vi "pumpPIDantiWindup_Filter.vi"(4 "Saturation U":dbl, 6 "Saturation M":dbl, 7 "Reset":bool, 8 "PID Gains":cluster{"Kp":dbl, "Kd":dbl, "Ki":dbl, "Ts":dbl}={"Kp"=0.0, "Kd"=0.0, "Ki"=0.0, "Ts"=1.0}, 10 "Feedback":dbl, 11 "Reference":dbl) -> (3 "Control":dbl)   [LabVIEW 2016]
uses:
  <vilib>/ptbypt/NI_PtbyPt.lvlib
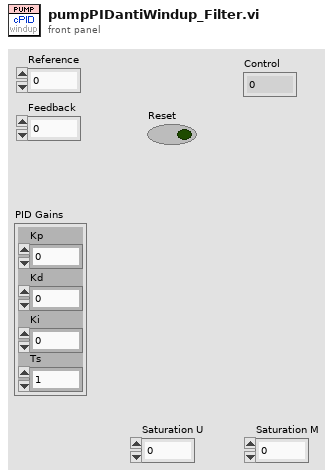
[diagram p1: front panel]
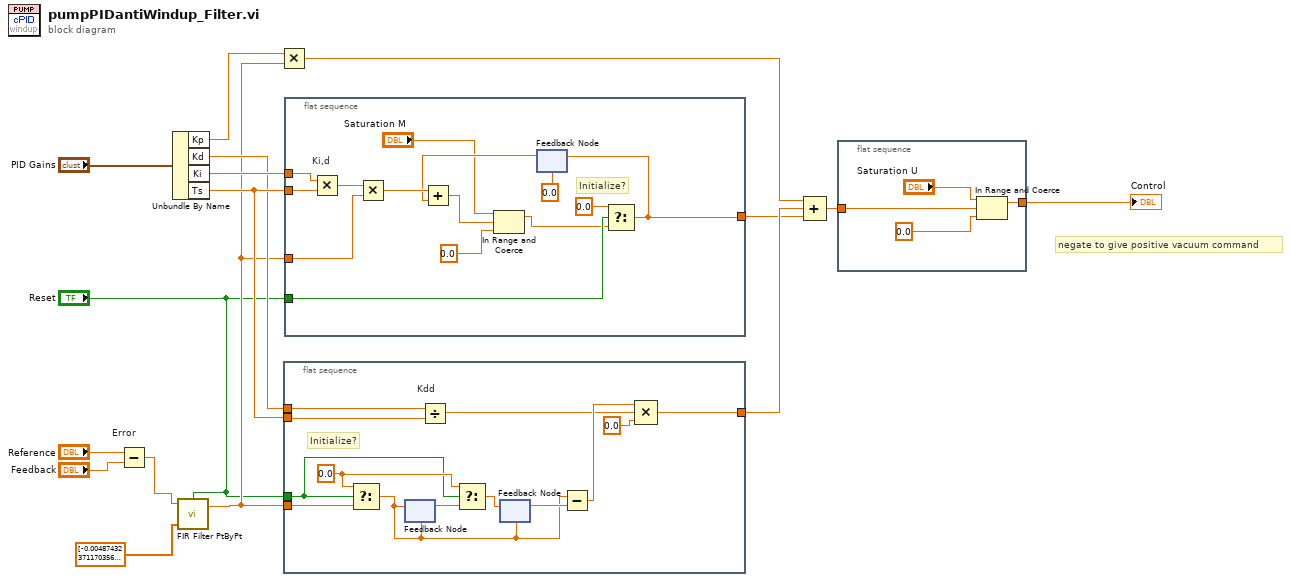
[diagram p0: block diagram]
diagram:
  # "negate to give positive vacuum command"
  n1 = Subtract "Error"(x="Reference", y="Feedback") -> (x-y=w4:dbl)
  n2 = Unbundle By Name("PID Gains") -> ("Kp"=w13:dbl, "Kd"=w7:dbl, "Ki"=w9:dbl, "Ts"=w8:dbl)
  n3 = call <vilib>:"FIR Filter PtByPt.vi"("initialize"="Reset", "Forward Coefficients"=dbl[] [-0.004874323711703563, 0.0002755179534692969, 0.00034979384442294123, 0.0004743306365063748, 0.0006455839849496639, 0.0008593421367122514, 0.0011105542954171345, 0.0013932008589386232, 0.0017002061146305755, 0.0020233938629409813, 0.0023534861364194965, 0.002680144717769675, 0.0029920545680283722, 0.0032770475851078484, 0.0035222643551458045, 0.0037143507658265328, 0.0038396855532291966, 0.0038846340822229256, 0.0038358229440492264, 0.0036804293206938884, 0.0034064785386602845, 0.0030031428364651626, 0.00246103411865547, 0.0017724833784128933, 0.0009317995504633908, -6.44991890842201e-05, -0.0012174882291962443, -0.002525679389453003, -0.003984909036538945, -0.005588275736641031, -0.007326130694600945, -0.009186123092035184, -0.011153301219469745, -0.013210269030471289, -0.015337396459345499, -0.017513080569872604, -0.019714053372687328, -0.021915730994624585, -0.02409259783453903, -0.026218618424399456, -0.02826766895646481, -0.03021397985794641, -0.03203258041031564, -0.033699736233084074, -0.035193370488060906, -0.03649345991099431, -0.03758239723888285, -0.038445312263475084, -0.03907034458975983, -0.03944886219298527, 0.9604243789749876, -0.03944886219298527, -0.03907034458975983, -0.038445312263475084, -0.03758239723888285, -0.03649345991099431, -0.035193370488060906, -0.033699736233084074, -0.03203258041031564, -0.03021397985794641, -0.02826766895646481, -0.026218618424399456, -0.02409259783453903, -0.021915730994624585, -0.019714053372687328, -0.017513080569872604, -0.015337396459345499, -0.013210269030471289, -0.011153301219469745, -0.009186123092035184, -0.007326130694600945, -0.005588275736641031, -0.003984909036538945, -0.002525679389453003, -0.0012174882291962443, -6.44991890842201e-05, 0.0009317995504633908, 0.0017724833784128933, 0.00246103411865547, 0.0030031428364651626, 0.0034064785386602845, 0.0036804293206938884, 0.0038358229440492264, 0.0038846340822229256, 0.0038396855532291966, 0.0037143507658265328, 0.0035222643551458045, 0.0032770475851078484, 0.0029920545680283722, 0.002680144717769675, 0.0023534861364194965, 0.0020233938629409813, 0.0017002061146305755, 0.0013932008589386232, 0.0011105542954171345, 0.0008593421367122514, 0.0006455839849496639, 0.0004743306365063748, 0.00034979384442294123, 0.0002755179534692969, -0.004874323711703563] ("num_HP"), "x"=w4) -> ("Filtered x"=w3:dbl)  [unwired: 1 in, 1 out]
  n4 = Multiply(x=w13, y=w3) -> (x*y=w12:dbl)
  n5 = flat-sequence {
    tunnel: [w26] -> w11
    tunnel: w3 -> [w21]
    tunnel: w8 -> [w25]
    tunnel: w7 -> [w24]
    tunnel: "Reset" -> [w17]
    frame #0 {
      w18 = 0.0 ("t")
      # "Initialize?"
      n6 = Select(t=w18, s=w17, f=w21) -> (s? t:f=w22:dbl)
      n7 = feedback #1(w22) -> (w20:dbl)
      n8 = feedback-in #1(w22) -> ()
      n9 = Divide "Kdd"(x=w24, y=w25) -> (x/y=w23:dbl)
      n10 = Select(t=w18, s=w17, f=w20) -> (s? t:f=w19:dbl)
      n11 = feedback #2(w22) -> (w29:dbl)
      n12 = feedback-in #2(w19) -> ()
      n13 = Subtract(x=w22, y=w29) -> (x-y=w28:dbl)
      n14 = Compound Arithmetic op=MULTIPLY(w28, w23, 0.0 ("value")) -> (w26:dbl)
    }
  }
  n15 = flat-sequence {
    tunnel: [w32] -> w10
    tunnel: w3 -> [w43]
    tunnel: w9 -> [w41]
    tunnel: w8 -> [w39]
    tunnel: "Reset" -> [w35]
    frame #0 {
      # "Initialize?"
      n16 = Multiply "Ki,d"(x=w41, y=w39) -> (x*y=w40:dbl)
      n17 = Multiply(x=w40, y=w43) -> (x*y=w42:dbl)
      n18 = feedback #3(0.0 ("value")) -> (w36:dbl)
      n19 = Add(x=w42, y=w36) -> (x+y=w38:dbl)
      n20 = In Range and Coerce(upper limit="Saturation M", x=w38, lower limit=0.0 ("upper limit")) -> (coerced(x)=w34:dbl)  [unwired: 1 out]
      n21 = Select(t=0.0 ("value"), s=w35, f=w34) -> (s? t:f=w32:dbl)
      n22 = feedback-in #3(w32) -> ()
    }
  }
  n23 = Compound Arithmetic op=ADD(w12, w11, w10) -> (w6:dbl)
  n24 = flat-sequence {
    tunnel: w6 -> [w47]
    tunnel: [w46] -> w5
    frame #0 {
      n25 = In Range and Coerce(upper limit="Saturation U", x=w47, lower limit=0.0 ("upper limit")) -> (coerced(x)=w46:dbl)  [unwired: 1 out]
    }
  }
  "Control" <- w5
